vi "FP ERD SendReceive Example.vi"() -> ()   [LabVIEW 2016]
uses:
  type defs/ERD Read Data In.ctl
  type defs/Data Type.ctl
  type defs/Source_Destination.ctl
  type defs/ERD Read Data Out.ctl
  library/GEA2_Toolkit.lvlib
panel:
  out "ERD Data Out":T1[](array[typedef]) {"ERD Number" format="%.0x"}
  out "Data":string[][](array[string])
  in  "stop":bool
  in  "Inverter Address":T2={"Source"=240, "Destination"=63} {"Destination" format="%.0x"; "Source" format="%.0x"}
  in  "2019 Inverter CMDs":T3[](array[typedef])=[{"ERD Number"=62218, "Data Type"=enum."string"}, {"ERD Number"=62229, "Data Type"=enum."string"}, {"ERD Number"=62224, "Data Type"=enum."string"}] {"ERD Number" format="%.0x"}
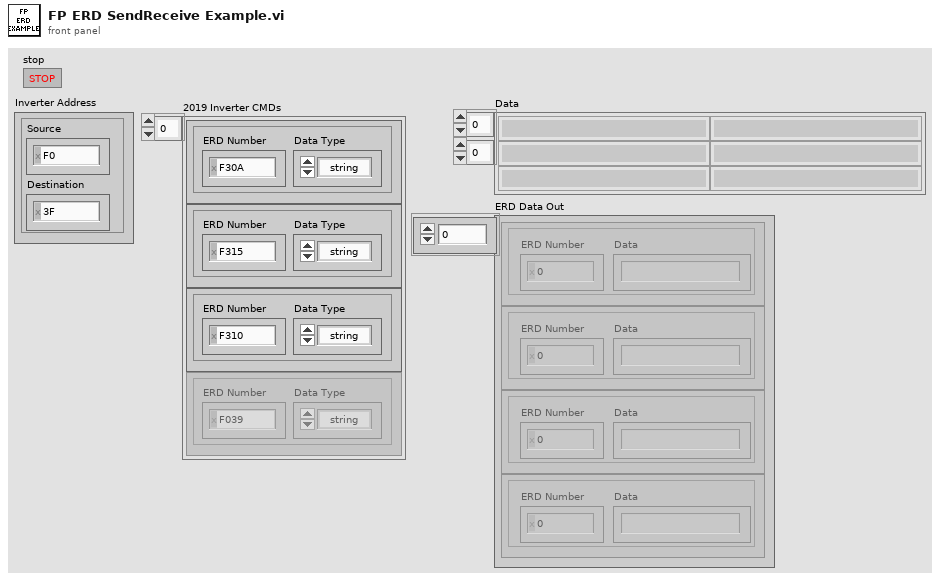
[diagram p1: front panel]
types:
  T1 = typedef "GEA2_Toolkit.lvlib/ERD Read Data Out.ctl" = cluster{"ERD Number":u16, "Data":string}
  T2 = typedef "GEA2_Toolkit.lvlib/Source_Destination.ctl" = cluster{"Source":u8, "Destination":u8}
  T3 = typedef "GEA2_Toolkit.lvlib/ERD Read Data In.ctl" = cluster{"ERD Number":u16, "Data Type":T4}
  T4 = typedef "GEA2_Toolkit.lvlib/Data Type.ctl" = enum16{"string", "boolean", "uint8_t", "uint16_t", "uint32_t", "uint64_t"}
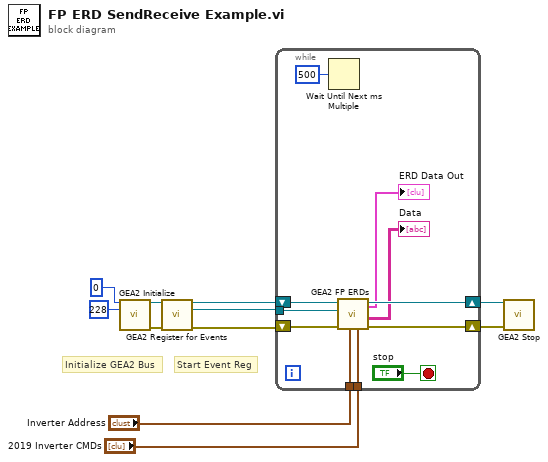
[diagram p0: block diagram]
diagram:
  # "Start Event Reg"
  # "Initialize GEA2 Bus"
  n1 = call "GEA2 Initialize.vi"("Board Index"=0, "Source Address"=u8 228) -> ("GEA2 Reference Out"=w11:refnum<k24>, "error out"=w10:errorcluster)  [unwired: 11 in, 1 out]
  n2 = call "GEA2 Register for Events.vi"("GEA2 Reference In"=w11, "Error In"=w10) -> ("GEA2 Reference Out"=w5:refnum<k24>, "GEA2 Event Registration"=w4:refnum<event-registration>, "Error Out"=w2:errorcluster)  [unwired: 11 in]
  n3 = while {
    tunnel: "2019 Inverter CMDs" -> [w22]
    tunnel: "Inverter Address" -> [w21]
    tunnel: w4 -> [w19]
    shift-right: [w18] -> w3
    shift-left: w5 -> [w20]
    shift-right: [w16] -> w1
    shift-left: w2 -> [w17]
    stop <- "stop" stop-if-true
    n4 = Wait Until Next ms Multiple(millisecond multiple=u32 500) -> ()  [unwired: 1 out]
    n5 = call "GEA2 FP ERDs.vi"("2019 Inverter CMDs"=w22, "Inverter Address"=w21, "Error In"=w17, "GEA2 Event Registration In"=w19, ".NET Refnum in"=w20) -> ("Error Out"=w16:errorcluster, "Data"=→"Data":string[][], ".NET Refnum out"=w18:refnum<k24>, "ERD Data Out"=→"ERD Data Out":T1[])  [unwired: 2 in, 1 out]
  }
  n6 = call "GEA2 Stop.vi"("GEA2 Reference Out"=w3, "Error In"=w1) -> ()  [unwired: 13 in, 1 out]
